vi "Digital IO.vi"(1 "DO 4":bool, 2 "DO 3":bool, 3 "DO in":bool, 4 "DO 1":bool) -> (0 "string":string)   [LabVIEW 2026]
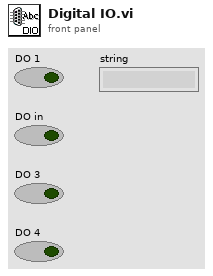
[diagram p1: front panel]
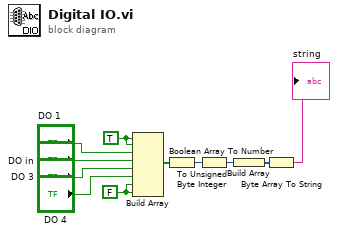
[diagram p0: block diagram]
diagram:
  w6 = FALSE
  w5 = TRUE
  n1 = Build Array(w5, w5, "DO 1", "DO in", "DO 3", "DO 4", w6, w6) -> (w7:bool[])
  n2 = Boolean Array To Number(Boolean array=w7) -> (number=w8:u32)
  n3 = To Unsigned Byte Integer(number=w8) -> (unsigned 8bit integer=w9:u8)
  n4 = Build Array(w9) -> (w10:u8[])
  n5 = Byte Array To String(unsigned byte array=w10) -> (string=→"string":string)
